vi "Render Misc.vi"(8 "error in (no error)":errorcluster, 11 "Main Controller Actor in":refnum<class "Main Controller Actor.lvclass">) -> (0 "error out":errorcluster)   [LabVIEW 2021, in "Main Controller Actor.lvclass"]
uses:
  Main Controller Actor.lvclass
  Player.ctl
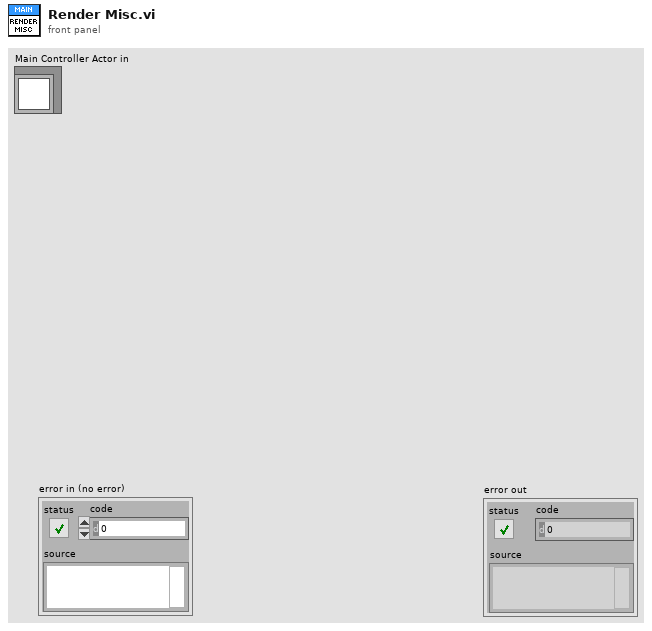
[diagram p1: front panel]
types:
  T1 = typedef "Main Controller Actor.lvclass/Player.ctl" = enum16{"1", "2"}
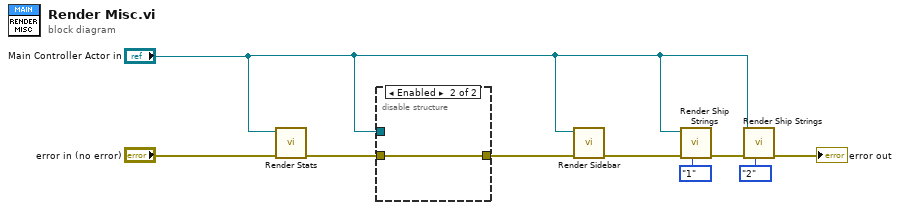
[diagram p0: block diagram]
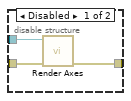
[diagram p2: hidden frame]
diagram:
  n1 = call "Render Stats.vi"("error in (no error)"="error in (no error)", "Main Controller Actor in"="Main Controller Actor in") -> ("error out"=w6:errorcluster)  [unwired: 8 in, 1 out]
  n2 = disable-structure shown="Enabled" {
    disable-tunnel: w6 -> [w12 w13]
    disable-tunnel: [w11 w13] -> w8
    disable-tunnel: "Main Controller Actor in" -> [w10 _]
    frame Disabled {
      n3 = call "Render Axes.vi"("error in (no error)"=w12, "Main Controller Actor in"=w10) -> ("error out"=w11:errorcluster)  [unwired: 9 in]
    }
    frame Enabled {
    }
  }
  n4 = call "Render Sidebar.vi"("error in (no error)"=w8, "Main Controller Actor in"="Main Controller Actor in") -> ("error out"=w7:errorcluster)  [unwired: 9 in]
  n5 = call "Render Ship Strings.vi"("Player"=Player."1", "error in (no error)"=w7, "Main Controller Actor in"="Main Controller Actor in") -> ("error out"=w4:errorcluster)  [unwired: 8 in]
  n6 = call "Render Ship Strings.vi"("Player"=Player."2", "error in (no error)"=w4, "Main Controller Actor in"="Main Controller Actor in") -> ("error out"=→"error out":errorcluster)  [unwired: 8 in]
